vi "tut_testing.vi"() -> ()   [LabVIEW 2023]
panel:
  out "String":string
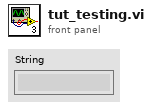
[diagram p1: front panel]
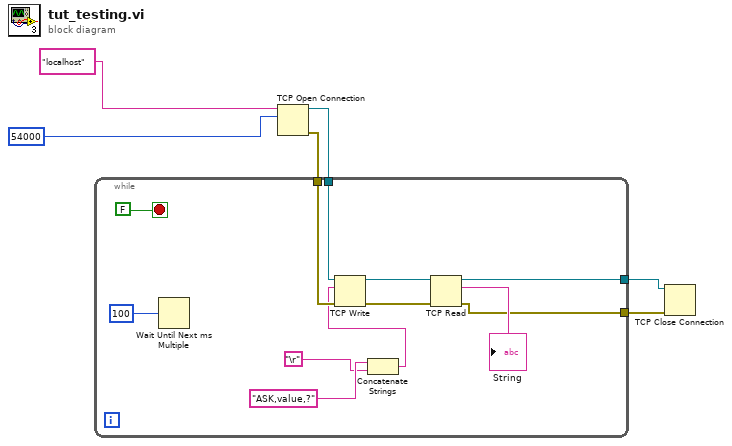
[diagram p0: block diagram]
diagram:
  n1 = TCP Open Connection(address="localhost", remote port or service name=54000) -> (connection ID=w1:refnum<k5>, error out=w2:errorcluster)  [unwired: 3 in]
  n2 = while {
    tunnel: [w15] -> w6
    tunnel: [w14] -> w5
    tunnel: w2 -> [w11]
    tunnel: w1 -> [w10]
    stop <- FALSE stop-if-true
    n3 = Wait Until Next ms Multiple(millisecond multiple=u32 100) -> ()  [unwired: 1 out]
    n4 = Concatenate Strings("ASK,value,?", "\r") -> (w7:string)
    n5 = TCP Write(connection ID=w10, data in=w7, error in (no error)=w11) -> (connection ID out=w16:refnum<k5>, error out=w17:errorcluster)  [unwired: 1 in, 1 out]
    n6 = TCP Read(connection ID=w16, error in (no error)=w17) -> (connection ID out=w15:refnum<k5>, data out=→"String":string, error out=w14:errorcluster)  [unwired: 3 in]
  }
  n7 = TCP Close Connection(connection ID=w6, error in (no error)=w5) -> ()  [unwired: 1 in, 2 out]
